vi "Actor.vi"(4 "Queue of Async Elements":refnum<queue>, 10 "Attributes":refnum<class "Attributes.lvclass">, 11 "TEMPLATE Actor in":refnum<class "TEMPLATE Actor.lvclass">) -> (0 "Error out":errorcluster, 3 "TEMPLATE Actor out":refnum<class "TEMPLATE Actor.lvclass">)   [LabVIEW 2025, in "_Template.lvlib" / "Templates.lvlib" / "TEMPLATE Actor.lvlib" / "TEMPLATE Actor.lvlib" / "TEMPLATE Actor.lvclass"]
uses:
  TEMPLATE Actor.lvclass
  C:/git/jettl/src/jettl/jettl/Actor/Actor.lvclass
  jettl/jettl/Attributes/Attributes.lvclass
  jettl/jettl/Async Elements.ctl
  TEMPLATE Refs/Refs.ctl
  TEMPLATE Actor.lvclass/TEMPLATE Actor.ctl
  C:/git/jettl/src/jettl Tools/_Template/Templates/TEMPLATE Actor/TEMPLATE Actor/TEMPLATE Actor/TEMPLATE Actor.lvclass
  TEMPLATE Refs/TEMPLATE Refs.lvlib
  jettl/jettl/jettl.lvlib
  jettl/jettl/Event Transport/Event Transport.lvlib
types:
  T1 = typedef "_Template.lvlib/Templates.lvlib/TEMPLATE Actor.lvlib/TEMPLATE Actor.lvlib/TEMPLATE Refs.lvlib/Refs.ctl" = cluster{"placeholder":refnum<vi>}
  T2 = cluster{"Msg Ref":refnum<event-registration>, "placeholder":refnum<event-registration>}
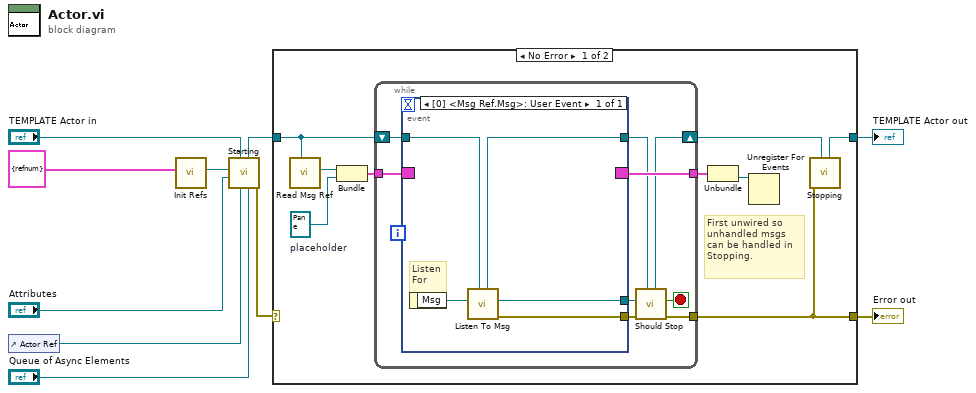
[diagram p0: block diagram]
diagram:
  n1 = control-ref of="Actor Ref"() -> (w1:refnum<vi>)
  n2 = call "Init Refs.vi"("Refs"=T1 {"placeholder"=refnum} ("Control Refs")) -> ("Refs"=w4:refnum<class "Refs.lvclass">)  [unwired: 10 in]
  n3 = call "Starting.vi"("Queue of Async Elements"="Queue of Async Elements", "Actor Ref"=w1, "Actor in"="TEMPLATE Actor in", "Attributes"="Attributes", "Refs"=w4) -> ("Error out"=w5:errorcluster, "Actor out"=w6:refnum<class "TEMPLATE Actor.lvclass">)  [unwired: 5 in]
  n4 = case shown="No Error" w5 {
    selector: w5 -> [_ w34]
    tunnel: [w17 w35] -> w9
    tunnel: w6 -> [w11 w35]
    tunnel: [w19 w34] -> w10
    frame No Error {
      w14 = refnum<event-registration> refnum  # placeholder
      # "First unwired so unhandled msgs can be handled in Stopping."
      n5 = call "Read Msg Ref.vi"("Actor"=w11) -> ("Msg Ref"=w12:refnum<event-registration>)  [unwired: 10 in]
      n6 = Bundle("Msg Ref"=w12, "placeholder"=w14) -> (w16:T2)  [unwired: 1 in]
      n7 = while {
        shift-right: [w21] -> w18
        shift-left: w11 -> [w27]
        tunnel: w16 -> [w28]
        tunnel: [w25] -> w19
        tunnel: [w22] -> w15
        stop <- w24 stop-if-true
        n8 = event shown="[0] <Msg Ref.Msg>: User Event" {
          selector: w28 -> [_]
          dyn-events: [_] -> w22
          timeout: _ -> [_]
          tunnel: w27 -> [w33]
          tunnel: [w31] -> w20
          tunnel: [w30] -> w26
          tunnel: [w29] -> w23
          event User Event {
            # "Listen\nFor"
            n9 = event-data() -> ("Msg"=w32:refnum<class "Msg.lvclass">)  [unwired: 1 in]
            n10 = call "Listen To Msg.vi"("Actor in"=w33, "Msg"=w32) -> ("Error out"=w30:errorcluster, "Msg Output"=w29:refnum<class "Msg Output.lvclass">, "Actor out"=w31:refnum<class "TEMPLATE Actor.lvclass">)  [unwired: 7 in]
          }
        }
        n11 = call "Should Stop.vi"("Actor in"=w20, "Error in"=w26, "Msg Output"=w23) -> ("Error out"=w25:errorcluster, "Stop"=w24:bool, "Actor out"=w21:refnum<class "TEMPLATE Actor.lvclass">)  [unwired: 6 in]
      }
      n12 = Unbundle(w15) -> ("placeholder"=w13:refnum<event-registration>)  [unwired: 1 out]
      n13 = Unregister For Events(event registration refnum=w13) -> ()  [unwired: 1 in, 1 out]
      n14 = call "Stopping.vi"("Actor in"=w18, "Error in"=w19) -> ("Actor out"=w17:refnum<class "TEMPLATE Actor.lvclass">)  [unwired: 9 in]
    }
    frame Error {
    }
  }
  "TEMPLATE Actor out" <- w9
  "Error out" <- w10
